vi "MFC_Steps.vi"() -> ()   [LabVIEW 2010]
uses:
  <vilib>/Utility/error.llb/DialogType.ctl
  <vilib>/DAQmx/write.llb/DAQmx Write (Analog DBL 1Chan 1Samp).vi
  <vilib>/DAQmx/create/channels.llb/DAQmx Create Channel (AO-Voltage-Basic).vi
  <vilib>/daqmx/miscellaneous.llb/DAQmx Fill In Error Info.vi
panel:
  out "Test in Progress...":bool
  in  "Voltage or SLPM":dbl[](array[numeric])
  in  "Conver to SLPM":bool
  out "Actual Vo":dbl[](array[numeric])
  in  "MFC Range (1,2,5,10 LPM)":dbl
  in  "Start Index":dbl
  out "current time":timestamp
  out "Voltage Output":dbl
  in  "stop":bool
  in  "Period (minutes)":dbl=30.0
  out "current time 2":timestamp
  out "x-y":dbl
  out "Countdown to next step":dbl
  out "Current Index":dbl
  in  "Go to next step":bool
  in  "Maximum Value":dbl=10.0 format="%0.2f"
  in  "Minimum Value":dbl=-10.0 format="%0.2f"
  in  "Physical Channel":tag="Dev1/ao0"
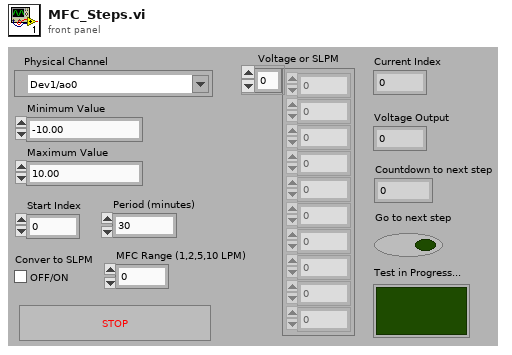
[diagram p1: front panel]
types:
  T1 = typedef "DialogType.ctl" = u16
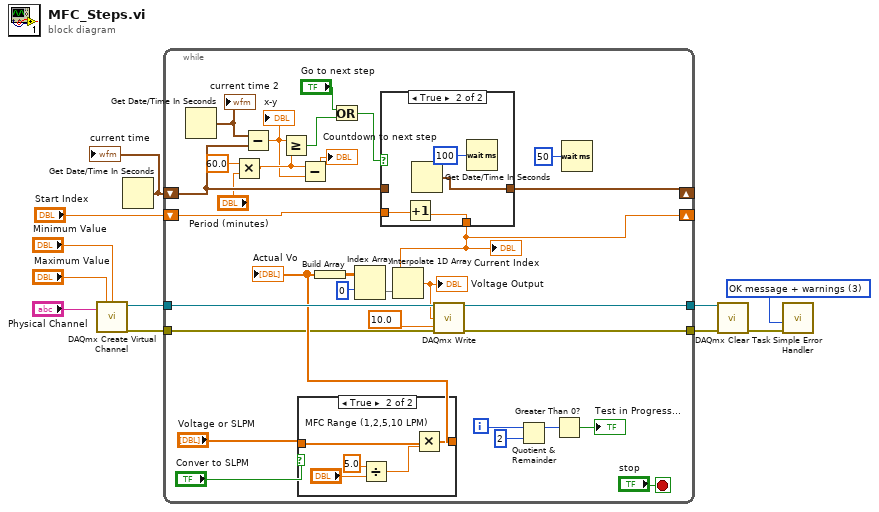
[diagram p0: block diagram]
diagram:
  w6 = T1 3 items=["no dialog", "OK message", "continue or stop message", "OK message + warnings", "continue/stop + warnings"] ("type of dialog (OK msg:1)")
  n1 = call-poly <vilib>:"DAQmx Create Virtual Channel.vi"("maximum value"="Maximum Value", "minimum value"="Minimum Value", "physical channels"="Physical Channel") -> ("task out"=w7:refnum<k21>, "error out"=w8:errorcluster)  [unwired: 11 in]
  n2 = Get Date/Time In Seconds() -> (seconds since 1Jan1904=w2:timestamp)
  "current time" <- w2
  n3 = while {
    tunnel: w8 -> [w16]
    tunnel: w7 -> [w42]
    tunnel: [w17] -> w5
    tunnel: [w41] -> w4
    shift-right: [w33] -> _
    shift-left: w2 -> [w32]
    shift-right: [w30] -> _
    shift-left: "Start Index" -> [w31]
    i -> [w13]
    stop <- "stop" stop-if-true
    n4 = Get Date/Time In Seconds() -> (seconds since 1Jan1904=w34:timestamp)
    "current time 2" <- w34
    n5 = Multiply(x=60.0, y="Period (minutes)") -> (x*y=w28:dbl)
    n6 = Subtract(x=w34, y=w32) -> (x-y=w20:dbl)
    "x-y" <- w20
    n7 = Greater Or Equal?(x=w20, y=w28) -> (x >= y?=w27:bool)
    n8 = case shown="True" "Conver to SLPM" {
      tunnel: [w43 w45] -> w21
      tunnel: "Voltage or SLPM" -> [w43 w44]
      frame False {
      }
      frame True {
        n9 = Divide(x=5.0, y="MFC Range (1,2,5,10 LPM)") -> (x/y=w46:dbl)
        n10 = Multiply(x=w44, y=w46) -> (x*y=w45:dbl[])
      }
    }
    "Actual Vo" <- w21
    n11 = Subtract(x=w28, y=w20) -> (x-y=→"Countdown to next step":dbl)
    n12 = Build Array(w21) -> (w39:dbl[][])
    n13 = Or(x="Go to next step", y=w27) -> (x .or. y?=w25:bool)
    n14 = Index Array(array=w39, index (row)=0) -> (element=w38:dbl[])  [unwired: 1 in]
    n15 = case shown="True" w25 {
      tunnel: w31 -> [w50 w54]
      tunnel: [w50 w53] -> w30
      tunnel: w32 -> [w49 _]
      tunnel: [w49 w52] -> w33
      frame False {
      }
      frame True {
        n16 = Increment(x=w54) -> (x+1=w53:dbl)
        n17 = Get Date/Time In Seconds() -> (seconds since 1Jan1904=w52:timestamp)
        n18 = Wait (ms)(milliseconds to wait=u32 100) -> ()  [unwired: 1 out]
      }
    }
    "Current Index" <- w30
    n19 = Interpolate 1D Array(1:w30, 2:w38) -> (0:w37:dbl)
    "Voltage Output" <- w37
    n20 = call-poly <vilib>:"DAQmx Write.vi"("task/channels in"=w42, "data"=w37, "timeout"=10.0, "error in"=w16) -> ("task out"=w41:refnum<k21>, "error out"=w17:errorcluster)  [unwired: 9 in, 1 out]
    n21 = Quotient & Remainder(x=w13, y=2) -> (x-y*floor(x/y)=w15:i32)  [unwired: 1 out]
    n22 = Greater Than 0?(x=w15) -> (x > 0?=→"Test in Progress...":bool)
    n23 = Wait (ms)(milliseconds to wait=u32 50) -> ()  [unwired: 1 out]
  }
  n24 = call <vilib>:"DAQmx Clear Task.vi"("task in"=w4, "error in"=w5) -> ("error out"=w3:errorcluster)  [unwired: 13 in]
  n25 = call <vilib>:"Simple Error Handler.vi"("type of dialog (OK msg:1)"=w6, "error in (no error)"=w3) -> ()  [unwired: 3 in, 5 out]
